vi "Assert Display Hinter.vi"() -> ()   [LabVIEW 2015, in "Member_Actor.lvlib" / "Member_Actor.lvclass"]
uses:
  Member_Actor.lvclass
  Member_Actor.lvclass/Member_Actor.ctl
panel:
  in  "String":string
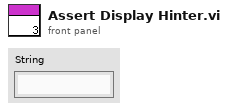
[diagram p1: front panel]
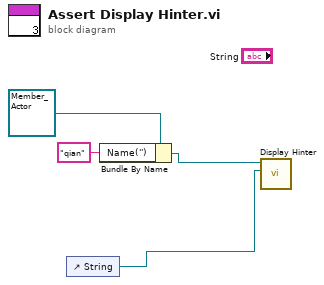
[diagram p0: block diagram]
diagram:
  n1 = control-ref of="String"() -> (w1:refnum<vi>)
  n2 = Bundle By Name(cluster=refnum<class "Member_Actor.lvclass"> refnum ("Member_Actor in"), "Name('')"="qian") -> (w2:refnum<class "Member_Actor.lvclass">)
  n3 = call "Display Hinter.vi"("Hint Ref"=w1, "Member_Actor in"=w2) -> ()  [unwired: 8 in, 2 out]
